vi "Config Paths.vi"(8 "error in (no error)":errorcluster) -> (0 "error out":errorcluster, 1 "Process Config":path, 3 "Global Config":path)   [LabVIEW 2020, in "MacroAssert.lvlib"]
uses:
  MacroAssert.lvlib
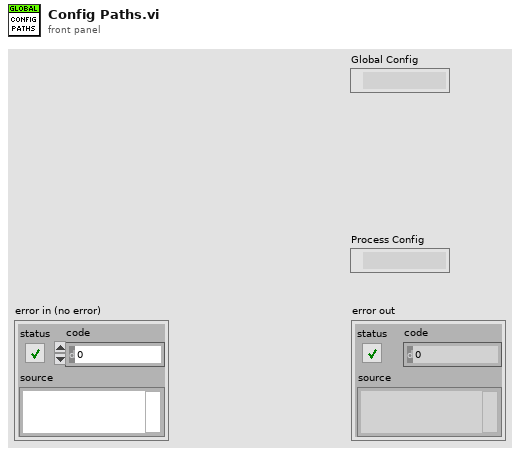
[diagram p1: front panel]
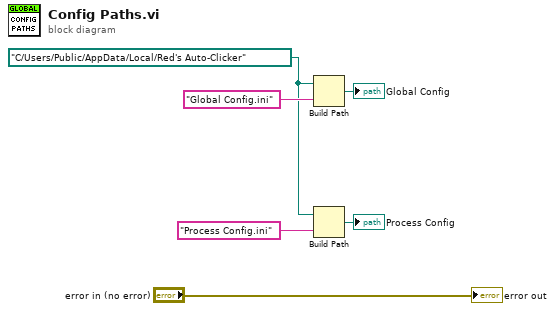
[diagram p0: block diagram]
diagram:
  w1 = path "C:/Users/Public/AppData/Local/Red's Auto-Clicker"
  n1 = Build Path(base path=w1, name or relative path="Global Config.ini") -> (appended path=→"Global Config":path)
  n2 = Build Path(base path=w1, name or relative path="Process Config.ini") -> (appended path=→"Process Config":path)
  "error out" <- "error in (no error)"
